vi "calcNoImgs.vi"(1 "filenames":string[](array[string]), 2 "regExp":string) -> (0 "noImgs":i32)   [LabVIEW 2015]
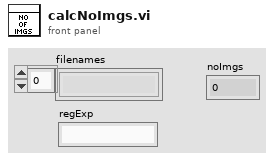
[diagram p1: front panel]
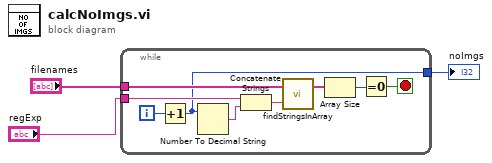
[diagram p0: block diagram]
diagram:
  n1 = while {
    tunnel: "filenames" -> [w10]
    tunnel: "regExp" -> [w11]
    tunnel: [w4] -> w1
    i -> [w5]
    stop <- w6 stop-if-true
    n2 = Increment(x=w5) -> (x+1=w4:i32)
    n3 = Number To Decimal String(number=w4) -> (decimal integer string=w12:string)  [unwired: 1 in]
    n4 = Concatenate Strings(w11, w12) -> (w9:string)
    n5 = call "findStringsInArray.vi"("Regular expression"=w9, "1D string array"=w10) -> ("Matched array"=w8:string[])  [unwired: 1 out]
    n6 = Array Size(array=w8) -> (size(s)=w7:i32)
    n7 = Equal To 0?(x=w7) -> (x = 0?=w6:bool)
  }
  "noImgs" <- w1
